vi "Read Image File.vi"   [LabVIEW 2020, in "image.lvlib"]
doc: "Read an Image file. A broad range of file formats are supported including jpeg, bitmap, png, webp, tiff and others."
uses:
  image.lvlib
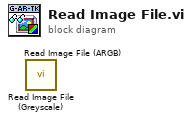
[diagram p0: block diagram]
diagram:
  n1 = call "Read Image File (Greyscale).vi"() -> ()  [unwired: 10 in, 2 out]
  n2 = call "Read Image File (ARGB).vi"() -> ()  [unwired: 10 in, 2 out]
